vi "RMM_4WIS_RT_DXs_V2_1team.vi"() -> ()   [LabVIEW 2019]
uses:
  <vilib>/Instr/_visa.llb/VISA Set IO Buffer Mask.ctl
  <vilib>/Instr/_visa.llb/VISA Flush IO Buffer Mask.ctl
  <vilib>/Instr/_visa.llb/VISA Configure Serial Port (Instr).vi
  <vilib>/FPGAPlugInAG/myRIO-1900/niLvFpga_Open_myRIO-1900.vi
  <vilib>/rvi/interface/common/dynamic/niFpgaDynamicAddResources.vi
  <vilib>/Utility/error.llb/Error Cluster From Error Code.vi
  <vilib>/rvi/errors/niLvFpgaAdjustHostInterfaceError.vi
  <vilib>/FPGAPlugInAG/Dynamic/niLvFpga_Close_Dynamic.vi
  <vilib>/rvi/interface/nirviOpenFPGA/nirviOpenFPGA.xnode
  FPGA Bitfiles/rmm4wisrobot_FPGATarget_RMM4WISFPGA_VGKxlyhi8sc.lvbitx
  RMM_4WIS_FPGA.vi
  <vilib>/rvi/interface/nirviReadWriteControl/nirviReadWriteControl.xnode
  <vilib>/rvi/interface/nirviCloseFPGA/nirviCloseFPGA.xnode
  <vilib>/rvi/interface/Simulation/niFpgaSimulationCallBeginRW.vi
  NiFpgaLv.dll
panel:
  out "RL_Steer_Feed(deg)":i16
  out "RR_Steer_Feed(deg)":i16
  out "FR_Steer_Feed(deg)":i16
  out "FL_Steer_Feed(deg)":i16
  out "HLV_M/A_Status":u8
  out "K_ZERO_CMD":T1
  out "RIO_Steer_Mode":u8
  out "HLV_NotAlive":bool
  out "HLV_E-Stop":bool
  out "RE_E-Stop":bool
  out "Re_M/A":bool
  out "FR_M1_Curr.MPS":dbl
  out "RL_M2_Curr.MPS":dbl
  out "RR_Steer_Feed":i16
  out "RL_Steer_Feed":i16
  out "FR_Steer_Feed":i16
  out "FL_Steer_Feed":i16
  out "Rear_Data":string
  out "RR_M1_Curr.RPM":i16
  out "RR_M1_Amp":u16
  out "RR_M1_Encoder":i32
  out "RR_M1_Staus":u8
  out "RL_M2_Curr.RPM":i16
  out "RL_M2_Amp":u16
  out "RL_M2_Staus":u8
  out "RL_M2_Encoder":i32
  out "RR_M1_Curr.MPS":dbl
  out "RL_RPM":i16
  out "R_TQ_Off":bool
  out "FL_M1_Curr.MPS":dbl
  out "FR_M2_Encoder":i32
  out "FR_M2_Staus":u8
  out "FR_M2_Amp":u16
  out "FR_M2_Curr.RPM":i16
  out "FL_M1_Staus":u8
  out "FR_RPM":i16
  out "FL_RPM":i16
  out "RR_RPM":i16
  out "FL_M1_Encoder":i32
  out "FL_M1_Amp":u16
  out "FL_M1_Curr.RPM":i16
  out "F_TQ_Off":bool
  out "Front_Data":string
  in  "정지":bool
  # "Front"
  # "Rear"
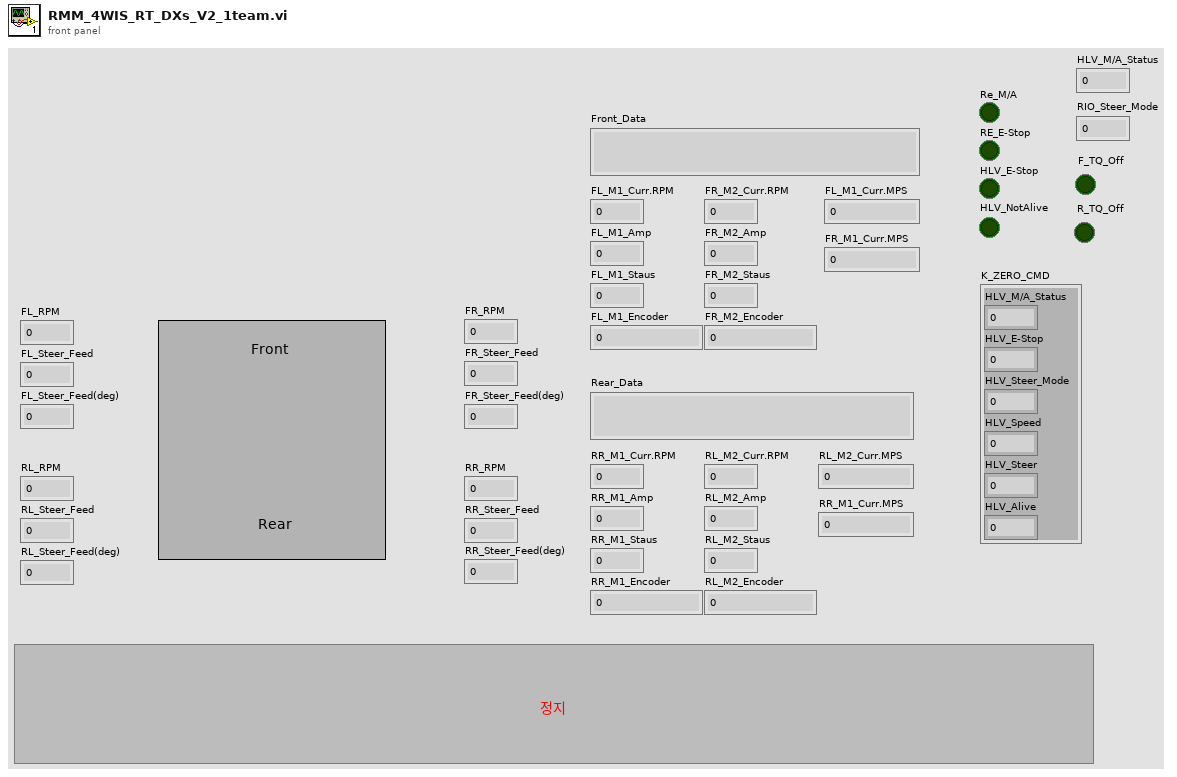
[diagram p1: front panel]
types:
  T1 = cluster{"HLV_M/A_Status":u8, "HLV_E-Stop":u8, "HLV_Steer_Mode":u8, "HLV_Speed":i16, "HLV_Steer":i16, "HLV_Alive":u8}
  T2 = cluster{"RIO_M/A_Status":u8, "RIO_E-Stop":u8, "RIO_Steer_Mode":u8, "RIO_FL_Speed":i16, "RIO_FL_Steer":i16, "RIO_Alive":u8, "RIO_FR_Speed":i16, "RIO_RL_Speed":i16, "RIO_RR_Speed":i16, "RIO_FR_Steer":i16, "RIO_RL_Steer":i16, "RIO_RR_Steer":i16}
  T3 = typedef "VISA Flush IO Buffer Mask.ctl" = u16
  T4 = typedef "VISA Set IO Buffer Mask.ctl" = u16
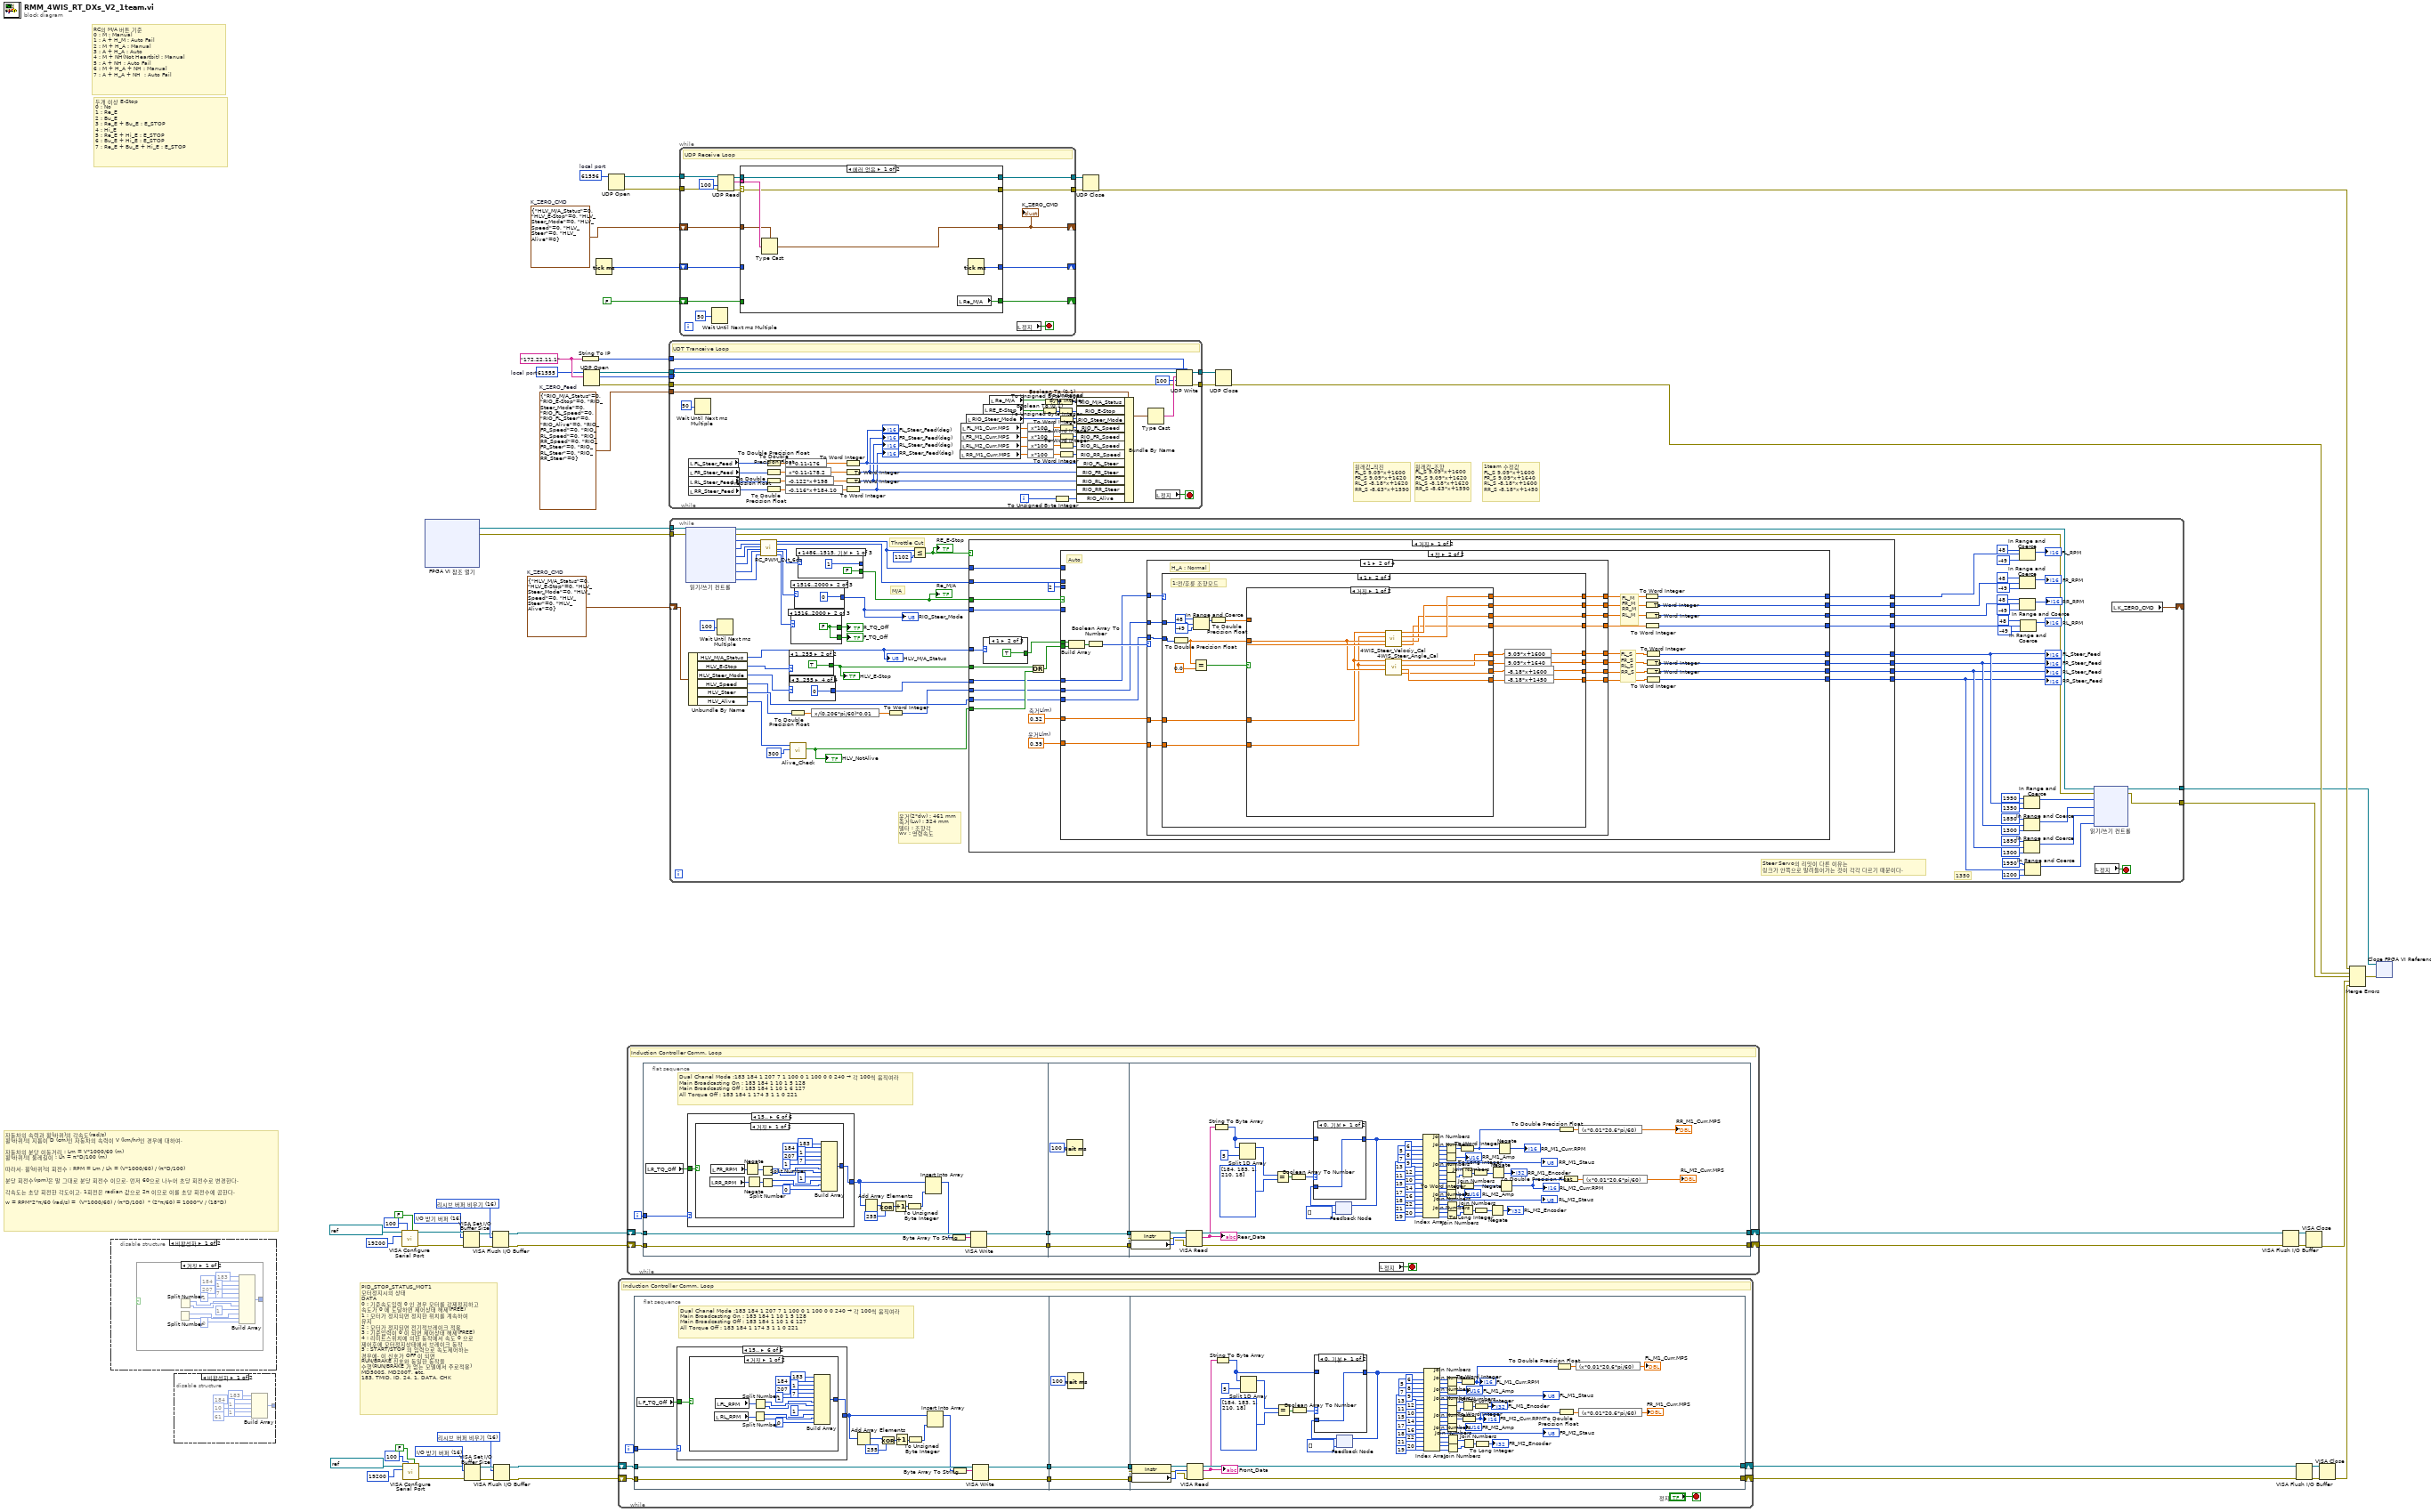
[diagram p0: block diagram]
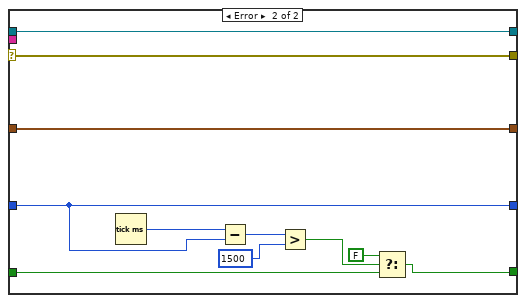
[diagram p2: hidden frame]
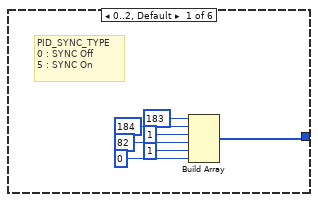
[diagram p3: hidden frame]
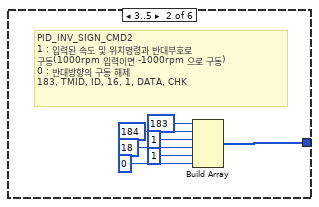
[diagram p4: hidden frame]
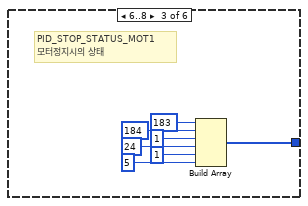
[diagram p5: hidden frame]
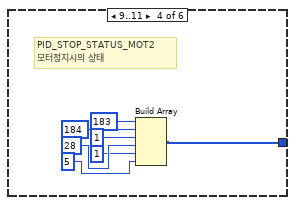
[diagram p6: hidden frame]
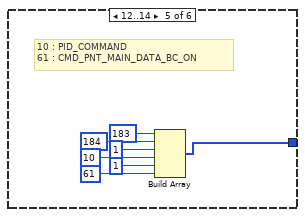
[diagram p7: hidden frame]
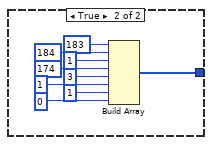
[diagram p8: hidden frame]
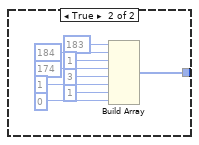
[diagram p11: hidden frame]
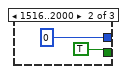
[diagram p13: hidden frame]
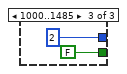
[diagram p14: hidden frame]
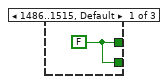
[diagram p15: hidden frame]
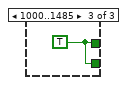
[diagram p16: hidden frame]
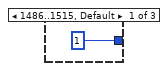
[diagram p17: hidden frame]
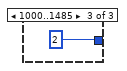
[diagram p18: hidden frame]
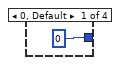
[diagram p19: hidden frame]
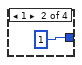
[diagram p20: hidden frame]
diagram:
  w3 = T2 {"RIO_M/A_Status"=0, "RIO_E-Stop"=0, "RIO_Steer_Mode"=0, "RIO_FL_Speed"=0, "RIO_FL_Steer"=0, "RIO_Alive"=0, "RIO_FR_Speed"=0, "RIO_RL_Speed"=0, "RIO_RR_Speed"=0, "RIO_FR_Steer"=0, "RIO_RL_Steer"=0, "RIO_RR_Steer"=0}  # K_ZERO_Feed
  w4 = T1 {"HLV_M/A_Status"=0, "HLV_E-Stop"=0, "HLV_Steer_Mode"=0, "HLV_Speed"=0, "HLV_Steer"=0, "HLV_Alive"=0}  # K_ZERO_CMD
  w12 = u16 61555  # local port
  w13 = "172.22.11.1" ("name")
  w21 = u16 61556  # local port
  w20 = T1 {"HLV_M/A_Status"=0, "HLV_E-Stop"=0, "HLV_Steer_Mode"=0, "HLV_Speed"=0, "HLV_Steer"=0, "HLV_Alive"=0}  # K_ZERO_CMD
  w35 = T3 16 items=["리시브 버퍼 비우기"=16, "전달 버퍼 디바이스에 쓰기"=32, "리시브 버퍼 비우기(I/O 없음)"=64, "전달 버퍼 비우기"=128] ("Mask")
  w34 = T4 16 items=["I/O 받기 버퍼"=16, "I/O 전달 버퍼"=32, "I/O 받기와 전달 버퍼"=48] ("Mask")
  w52 = T3 16 items=["리시브 버퍼 비우기"=16, "전달 버퍼 디바이스에 쓰기"=32, "리시브 버퍼 비우기(I/O 없음)"=64, "전달 버퍼 비우기"=128] ("Mask")
  w53 = T4 16 items=["I/O 받기 버퍼"=16, "I/O 전달 버퍼"=32, "I/O 받기와 전달 버퍼"=48] ("Mask")
  # "원래값_직진\nFL_S 9.09*x+1600\nFR_S 9.09*x+1620\nRL_S -8.18*x+1620\nRR_S -8.63*x+1590"
  # "1team 수정값\nFL_S 9.09*x+1600\nFR_S 9.09*x+1640\nRL_S -8.18*x+1600\nRR_S -8.18*x+1450"
  # "원래값_조향\nFL_S 9.09*x+1600\nFR_S 9.09*x+1620\nRL_S -8.18*x+1620\nRR_S -8.63*x+1590"
  # "PID_STOP_STATUS_MOT1\n모터정지시의 상태\nDATA\n0 : 기준속도입력 0 인 경우 모터를 강제정지하고\n속도가 0 에 도달하면 제어상태 해제(FREE)\n1 : 모터가 정지되면 정지한 위치를 계속하여\n유지\n2 : 모터가 정지되면 전기적브레이크 적용\n3 : 기준입력이 0 이 되면 제어상태 해제(FREE)\n4 : 리미트스위치에 의한 동작에서 속도 0 으로\n제어후에 모터정지상태에서 브레이크 동작\n5 : START/STOP 의 입력으로 속도제어하는\n경우에, 이 신호가 OFF 이 되면\nRUN/BRAKE 신호와 동일한 동작을\n수행(RUN/BRAKE 가 없는 모델에서 주로적용)\nMD500S, MD200T, etc.\n183, TMID, ID, 24, 1, DATA, CHK"
  # "두개 이상 E-Stop\n0 : No\n1 : Re_E\n2 : Bu_E\n3 : Re_E + Bu_E : E_STOP\n4 : Hi_E\n5 : Re_E + Hi_E : E_STOP\n6 : Bu_E + Hi_E : E_STOP\n7 : Re_E + Bu_E + Hi_E : E_STOP"
  # "RC의 M/A 버튼 기준\n0 : M : Manual \n1 : A + H_M : Auto Fail\n2 : M + H_A : Manual\n3 : A + H_A : Auto\n4 : M + NH(Not Heartbit) : Manual\n5 : A + NH : Auto Fail\n6 : M + H_A + NH : Manual\n7 : A + H_A + NH  : Auto Fail"
  # "자동차의 속력과 휠(바퀴)의 각속도(rad/s)\n휠(바퀴)의 지름이 D (cm)인 자동차의 속력이 V (km/hr)인 경우에 대하여,  \n\n자동차의 분당 이동거리 : Lm = V*1000/60 (m)  \n휠(바퀴)의 둘레길이 : Lh = π*D/100 (m)  \n\n따라서, 휠(바퀴)의 회전수 : RPM = Lm / Lh = (V*1000/60) / (π*D/100)  \n\n분당 회전수(rpm)은 말 그대로 분당 회전수 이므로, 먼저 60으로 나누어 초당 회전수로 변경한다.  \n\n각속도는 초당 회전한 각도이고, 1회전은 radian 값으로 2π 이므로 이를 초당 회전수에 곱한다.  \n\nw = RPM*2*π/60 (rad/s) =  (V*1000/60) / (π*D/100)  * (2*π/60) = 1000*V / (18*D)"
  n1 = disable-structure shown="비활성화" {
    frame Disabled {
      n2 = case shown="거짓" {
        selector: _ -> [_ _]
        tunnel: [w64 w73] -> _
        frame False {
          n3 = Split Number() -> (hi(x)=w61:u16, lo(x)=w60:u16)  [unwired: 1 in]
          n4 = Split Number() -> (hi(x)=w63:u16, lo(x)=w62:u16)  [unwired: 1 in]
          n5 = Build Array(u8 183, u8 184, u8 1, u8 207, u8 7, u8 1, w62, w63, u8 1, w60, w61, u8 0) -> (w64:u8[])
        }
        frame True {
          n6 = Build Array(u8 183, u8 184, u8 1, u8 174, u8 3, u8 1, u8 1, u8 0) -> (w73:u8[])
        }
      }
    }
    frame Enabled {
    }
  }
  n7 = disable-structure shown="비활성화" {
    disable-tunnel: [w88 _] -> _
    frame Disabled {
      n8 = Build Array(u8 183, u8 184, u8 1, u8 10, u8 1, u8 61) -> (w88:u8[])
    }
    frame Enabled {
    }
  }
  n9 = call-poly "VISA Configure Serial Port"("VISA resource name"=refnum<visa-resource-name> "ASRL2::INSTR", "timeout (10sec)"=u32 100, "Enable Termination\nChar (T)"=FALSE ("Enable Termination\nChar (T)"), "baud rate (9600)"=u32 19200) -> ("VISA resource name out"=w42:refnum<visa-resource-name>, "error out"=w43:errorcluster)  [unwired: 10 in]
  n10 = call-poly "VISA Configure Serial Port"("VISA resource name"=refnum<visa-resource-name> "ASRL1::INSTR", "timeout (10sec)"=u32 100, "Enable Termination\nChar (T)"=FALSE ("Enable Termination\nChar (T)"), "baud rate (9600)"=u32 19200) -> ("VISA resource name out"=w45:refnum<visa-resource-name>, "error out"=w44:errorcluster)  [unwired: 10 in]
  n11 = xnode "FPGA VI 참조 열기"() -> ("FPGA VI 참조 출력"=w2:refnum<k20>, "에러 출력"=w1:errorcluster)  [unwired: 2 in]
  n12 = VISA Set I/O Buffer Size(VISA resource name=w42, mask (16)=w34, error in (no error)=w43) -> (VISA resource name out=w32:refnum<visa-resource-name>, error out=w33:errorcluster)  [unwired: 1 in]
  n13 = VISA Set I/O Buffer Size(VISA resource name=w45, mask (16)=w53, error in (no error)=w44) -> (VISA resource name out=w55:refnum<visa-resource-name>, error out=w54:errorcluster)  [unwired: 1 in]
  n14 = VISA Flush I/O Buffer(VISA resource name=w32, mask (16)=w35, error in (no error)=w33) -> (VISA resource name out=w36:refnum<visa-resource-name>, error out=w37:errorcluster)
  n15 = VISA Flush I/O Buffer(VISA resource name=w55, mask (16)=w52, error in (no error)=w54) -> (VISA resource name out=w51:refnum<visa-resource-name>, error out=w50:errorcluster)
  n16 = String To IP(1:w13) -> (0:w14:u32)
  n17 = UDP Open(10:w13, 11:w12) -> (port=w15:refnum<k16>, 0:w16:errorcluster, 2:w17:u16)  [unwired: 3 in]
  n18 = Tick Count (ms)() -> (millisecond timer value=w24:u32)
  n19 = UDP Open(11:w21) -> (port=w22:refnum<k16>, 0:w23:errorcluster)  [unwired: 4 in, 1 out]
  n20 = while {
    shift-right: [w91] -> w49
    shift-left: w51 -> [w97]
    shift-right: [w90] -> w48
    shift-left: w50 -> [w96]
    i -> [w89]
    stop <- "정지" stop-if-true
    # "Induction Controller Comm. Loop"
    n21 = flat-sequence {
      tunnel: [w110] -> w94
      tunnel: [w109] -> w92
      tunnel: w97 -> [w112]
      tunnel: w96 -> [w111]
      tunnel: w89 -> [w107]
      tunnel: [w176] -> w95
      tunnel: w94 -> [w176]
      tunnel: [w175] -> w93
      tunnel: w92 -> [w175]
      tunnel: w95 -> [w245]
      tunnel: w93 -> [w244]
      tunnel: [w247] -> w91
      tunnel: [w246] -> w90
      frame #0 {
        # "Dual Chanel Mode :183 184 1 207 7 1 100 0 1 100 0 0 240 → 각 100씩 움직여라\nMain Broadcasting On : 183 184 1 10 1 5 128\nMain Broadcasting Off : 183 184 1 10 1 6 127\nAll Torque Off : 183 184 1 174 3 1 1 0 221"
        n22 = local read "F_TQ_Off"() -> (w99:bool)
        n23 = case shown="15.." w107 {
          tunnel: [w113 w120 w127 w134 w141 w149] -> w100
          tunnel: w99 -> [_ _ _ _ _ w148]
          frame 0..2, Default {
            # "PID_SYNC_TYPE\n0 : SYNC Off\n5 : SYNC On"
            n24 = Build Array(u8 183, u8 184, u8 1, u8 82, u8 1, u8 0) -> (w113:u8[])
          }
          frame 3..5 {
            # "PID_INV_SIGN_CMD2\n1 : 모터 2 에 관한 명령으로 입력된 속도 및\n위치명령과 반대부호로 구동\n(1000rpm 입력이면 -1000rpm 으로 구동)\n0 : 반대방향의 구동 해제"
            n25 = Build Array(u8 183, u8 184, u8 1, u8 18, u8 1, u8 0) -> (w120:u8[])
          }
          frame 6..8 {
            # "PID_STOP_STATUS_MOT1\n모터정지시의 상태"
            n26 = Build Array(u8 183, u8 184, u8 1, u8 24, u8 1, u8 5) -> (w127:u8[])
          }
          frame 9..11 {
            # "PID_STOP_STATUS_MOT2\n모터정지시의 상태"
            n27 = Build Array(u8 183, u8 184, u8 1, u8 28, u8 1, u8 5) -> (w134:u8[])
          }
          frame 12..14 {
            # "10 : PID_COMMAND\n61 : CMD_PNT_MAIN_DATA_BC_ON"
            n28 = Build Array(u8 183, u8 184, u8 1, u8 10, u8 1, u8 61) -> (w141:u8[])
          }
          frame 15.. {
            n29 = case shown="거짓" w148 {
              tunnel: [w156 w165] -> w149
              frame False {
                n30 = local read "RL_RPM"() -> (w150:i16)
                n31 = local read "FL_RPM"() -> (w151:i16)
                n32 = Split Number(x=w150) -> (hi(x)=w153:u8, lo(x)=w152:u8)
                n33 = Split Number(x=w151) -> (hi(x)=w155:u8, lo(x)=w154:u8)
                n34 = Build Array(u8 183, u8 184, u8 1, u8 207, u8 7, u8 1, w154, w155, u8 1, w152, w153, u8 0) -> (w156:u8[])
              }
              frame True {
                n35 = Build Array(u8 183, u8 184, u8 1, u8 174, u8 3, u8 1, u8 1, u8 0) -> (w165:u8[])
              }
            }
          }
        }
        n36 = Add Array Elements(numeric array=w100) -> (sum=w104:u8)
        n37 = Exclusive Or(1:u8 255 ("y"), 2:w104) -> (0:w105:u8)
        n38 = Increment(x=w105) -> (x+1=w106:u8)
        n39 = To Unsigned Byte Integer(number=w106) -> (unsigned 8bit integer=w102:u8)
        n40 = Insert Into Array(array=w100, new element=w102) -> (w101:u8[])  [unwired: 1 in]
        n41 = Byte Array To String(unsigned byte array=w101) -> (string=w108:string)
        n42 = VISA Write(VISA resource name=w112, write buffer=w108, error in (no error)=w111) -> (VISA resource name out=w110:refnum<visa-resource-name>, error out=w109:errorcluster)  [unwired: 1 out]
      }
      frame #1 {
        n43 = Wait (ms)(milliseconds to wait=u32 100 ("대기 시간 (ms)")) -> ()  [unwired: 1 out]
      }
      frame #2 {
        n44 = property class="Instr"(reference=w245, error in=w244) -> (reference out=w243:refnum<visa-resource-name>, error out=w241:errorcluster, "Serial Settings:Number of Bytes at Serial Port"=w242:u32)
        n45 = VISA Read(VISA resource name=w243, byte count=w242, error in (no error)=w241) -> (VISA resource name out=w247:refnum<visa-resource-name>, read buffer=w240:string, error out=w246:errorcluster)  [unwired: 1 out]
        "Front_Data" <- w240
        n46 = String To Byte Array(string=w240) -> (unsigned byte array=w239:u8[])
        n47 = Split 1D Array(array=w239, index=5) -> (first subarray=w235:u8[])  [unwired: 1 out]
        n48 = Equal?(x=w235, y=u8[] [184, 183, 1, 210, 18]) -> (x = y?=w237:bool[])
        n49 = Boolean Array To Number(Boolean array=w237) -> (number=w236:u32)
        n50 = feedback #1(u8[] [] ("unsigned byte array")) -> (w183:u8[])
        n51 = case shown="0, 기본" w236 {
          tunnel: w239 -> [_ w249]
          tunnel: [w248 w249] -> w184
          tunnel: w183 -> [w248 _]
          frame 0, Default {
          }
          frame 31 {
          }
        }
        n52 = feedback-in #1(w184) -> ()
        n53 = Index Array(array=w184, index #1=6, index #2=5, index #3=8, index #4=7, index #5=9, index #6=13, index #7=12, index #8=11, index #9=10, index #10=15, index #11=14, index #12=17, index #13=16, index #14=18, index #15=22, index #16=21, index #17=20, index #18=19) -> (element #1=w232:u8, element #2=w231:u8, element #3=w229:u8, element #4=w227:u8, element #5=→"FL_M1_Staus":u8, element #6=w226:u8, element #7=w225:u8, element #8=w224:u8, element #9=w223:u8, element #10=w217:u8, element #11=w216:u8, element #12=w214:u8, element #13=w213:u8, element #14=→"FR_M2_Staus":u8, element #15=w207:u8, element #16=w206:u8, element #17=w205:u8, element #18=w204:u8)
        n54 = Join Numbers(hi=w232, lo=w231) -> ((hi.lo)=w230:u16)
        n55 = Join Numbers(hi=w229, lo=w227) -> ((hi.lo)=→"FL_M1_Amp":u16)
        n56 = Join Numbers(hi=w226, lo=w225) -> ((hi.lo)=w219:u16)
        n57 = Join Numbers(hi=w224, lo=w223) -> ((hi.lo)=w218:u16)
        n58 = Join Numbers(hi=w217, lo=w216) -> ((hi.lo)=w215:u16)
        n59 = Join Numbers(hi=w214, lo=w213) -> ((hi.lo)=→"FR_M2_Amp":u16)
        n60 = Join Numbers(hi=w207, lo=w206) -> ((hi.lo)=w210:u16)
        n61 = Join Numbers(hi=w205, lo=w204) -> ((hi.lo)=w203:u16)
        n62 = To Word Integer(number=w230) -> (16bit integer=w182:i16)
        "FL_M1_Curr.RPM" <- w182
        n63 = Join Numbers(hi=w219, lo=w218) -> ((hi.lo)=w222:u32)
        n64 = To Word Integer(number=w215) -> (16bit integer=w177:i16)
        "FR_M2_Curr.RPM" <- w177
        n65 = Join Numbers(hi=w210, lo=w203) -> ((hi.lo)=w208:u32)
        n66 = To Long Integer(number=w222) -> (32bit integer=→"FL_M1_Encoder":i32)
        n67 = To Long Integer(number=w208) -> (32bit integer=→"FR_M2_Encoder":i32)
        n68 = To Double Precision Float(number=w182) -> (double precision float=w180:dbl)
        n69 = To Double Precision Float(number=w177) -> (double precision float=w179:dbl)
        n70 = expression code="(x*0.01*20.6*pi/60)"(w180) -> (→"FL_M1_Curr.MPS":dbl)
        n71 = expression code="(x*0.01*20.6*pi/60)"(w179) -> (→"FR_M1_Curr.MPS":dbl)
      }
    }
  }
  n72 = while {
    shift-right: [w253] -> w38
    shift-left: w36 -> [w259]
    shift-right: [w252] -> w39
    shift-left: w37 -> [w258]
    i -> [w251]
    stop <- w250 stop-if-true
    # "Induction Controller Comm. Loop"
    n73 = flat-sequence {
      tunnel: [w271] -> w256
      tunnel: [w270] -> w254
      tunnel: w259 -> [w273]
      tunnel: w258 -> [w272]
      tunnel: w251 -> [w268]
      tunnel: [w339] -> w257
      tunnel: w256 -> [w339]
      tunnel: [w338] -> w255
      tunnel: w254 -> [w338]
      tunnel: w257 -> [w412]
      tunnel: w255 -> [w411]
      tunnel: [w414] -> w253
      tunnel: [w413] -> w252
      frame #0 {
        # "Dual Chanel Mode :183 184 1 207 7 1 100 0 1 100 0 0 240 → 각 100씩 움직여라\nMain Broadcasting On : 183 184 1 10 1 5 128\nMain Broadcasting Off : 183 184 1 10 1 6 127\nAll Torque Off : 183 184 1 174 3 1 1 0 221"
        n74 = local read "R_TQ_Off"() -> (w260:bool)
        n75 = case shown="15.." w268 {
          tunnel: [w274 w281 w288 w295 w302 w310] -> w261
          tunnel: w260 -> [_ _ _ _ _ w309]
          frame 0..2, Default {
            # "PID_SYNC_TYPE\n0 : SYNC Off\n5 : SYNC On"
            n76 = Build Array(u8 183, u8 184, u8 1, u8 82, u8 1, u8 0) -> (w274:u8[])
          }
          frame 3..5 {
            # "PID_INV_SIGN_CMD2\n1 : 입력된 속도 및 위치명령과 반대부호로\n구동(1000rpm 입력이면 -1000rpm 으로 구동)\n0 : 반대방향의 구동 해제\n183, TMID, ID, 16, 1, DATA, CHK"
            n77 = Build Array(u8 183, u8 184, u8 1, u8 18, u8 1, u8 0) -> (w281:u8[])
          }
          frame 6..8 {
            # "PID_STOP_STATUS_MOT1\n모터정지시의 상태"
            n78 = Build Array(u8 183, u8 184, u8 1, u8 24, u8 1, u8 5) -> (w288:u8[])
          }
          frame 9..11 {
            # "PID_STOP_STATUS_MOT2\n모터정지시의 상태"
            n79 = Build Array(u8 183, u8 184, u8 1, u8 28, u8 1, u8 5) -> (w295:u8[])
          }
          frame 12..14 {
            # "10 : PID_COMMAND\n61 : CMD_PNT_MAIN_DATA_BC_ON"
            n80 = Build Array(u8 183, u8 184, u8 1, u8 10, u8 1, u8 61) -> (w302:u8[])
          }
          frame 15.. {
            n81 = case shown="거짓" w309 {
              tunnel: [w319 w328] -> w310
              frame False {
                n82 = local read "RR_RPM"() -> (w314:i16)
                n83 = local read "FR_RPM"() -> (w313:i16)
                n84 = Negate(x=w313) -> (-x=w312:i16)
                n85 = Negate(x=w314) -> (-x=w311:i16)
                n86 = Split Number(x=w311) -> (hi(x)=w316:u8, lo(x)=w315:u8)
                n87 = Split Number(x=w312) -> (hi(x)=w318:u8, lo(x)=w317:u8)
                n88 = Build Array(u8 183, u8 184, u8 1, u8 207, u8 7, u8 1, w317, w318, u8 1, w315, w316, u8 0) -> (w319:u8[])
              }
              frame True {
                n89 = Build Array(u8 183, u8 184, u8 1, u8 174, u8 3, u8 1, u8 1, u8 0) -> (w328:u8[])
              }
            }
          }
        }
        n90 = Add Array Elements(numeric array=w261) -> (sum=w265:u8)
        n91 = Exclusive Or(1:u8 255 ("y"), 2:w265) -> (0:w266:u8)
        n92 = Increment(x=w266) -> (x+1=w267:u8)
        n93 = To Unsigned Byte Integer(number=w267) -> (unsigned 8bit integer=w263:u8)
        n94 = Insert Into Array(array=w261, new element=w263) -> (w262:u8[])  [unwired: 1 in]
        n95 = Byte Array To String(unsigned byte array=w262) -> (string=w269:string)
        n96 = VISA Write(VISA resource name=w273, write buffer=w269, error in (no error)=w272) -> (VISA resource name out=w271:refnum<visa-resource-name>, error out=w270:errorcluster)  [unwired: 1 out]
      }
      frame #1 {
        n97 = Wait (ms)(milliseconds to wait=u32 100 ("대기 시간 (ms)")) -> ()  [unwired: 1 out]
      }
      frame #2 {
        n98 = property class="Instr"(reference=w412, error in=w411) -> (reference out=w410:refnum<visa-resource-name>, error out=w408:errorcluster, "Serial Settings:Number of Bytes at Serial Port"=w409:u32)
        n99 = VISA Read(VISA resource name=w410, byte count=w409, error in (no error)=w408) -> (VISA resource name out=w414:refnum<visa-resource-name>, read buffer=w407:string, error out=w413:errorcluster)  [unwired: 1 out]
        "Rear_Data" <- w407
        n100 = String To Byte Array(string=w407) -> (unsigned byte array=w406:u8[])
        n101 = Split 1D Array(array=w406, index=5) -> (first subarray=w402:u8[])  [unwired: 1 out]
        n102 = Equal?(x=w402, y=u8[] [184, 183, 1, 210, 18]) -> (x = y?=w404:bool[])
        n103 = Boolean Array To Number(Boolean array=w404) -> (number=w403:u32)
        n104 = feedback #2(u8[] [] ("unsigned byte array")) -> (w352:u8[])
        n105 = case shown="0, 기본" w403 {
          tunnel: w406 -> [_ w416]
          tunnel: [w415 w416] -> w353
          tunnel: w352 -> [w415 _]
          frame 0, Default {
          }
          frame 31 {
          }
        }
        n106 = feedback-in #2(w353) -> ()
        n107 = Index Array(array=w353, index #1=6, index #2=5, index #3=8, index #4=7, index #5=9, index #6=13, index #7=12, index #8=11, index #9=10, index #10=15, index #11=14, index #12=17, index #13=16, index #14=18, index #15=22, index #16=21, index #17=20, index #18=19) -> (element #1=w399:u8, element #2=w398:u8, element #3=w396:u8, element #4=w394:u8, element #5=→"RR_M1_Staus":u8, element #6=w393:u8, element #7=w392:u8, element #8=w391:u8, element #9=w390:u8, element #10=w385:u8, element #11=w384:u8, element #12=w382:u8, element #13=w381:u8, element #14=→"RL_M2_Staus":u8, element #15=w376:u8, element #16=w375:u8, element #17=w374:u8, element #18=w373:u8)
        n108 = Join Numbers(hi=w399, lo=w398) -> ((hi.lo)=w397:u16)
        n109 = Join Numbers(hi=w396, lo=w394) -> ((hi.lo)=→"RR_M1_Amp":u16)
        n110 = Join Numbers(hi=w393, lo=w392) -> ((hi.lo)=w387:u16)
        n111 = Join Numbers(hi=w391, lo=w390) -> ((hi.lo)=w386:u16)
        n112 = Join Numbers(hi=w385, lo=w384) -> ((hi.lo)=w383:u16)
        n113 = Join Numbers(hi=w382, lo=w381) -> ((hi.lo)=→"RL_M2_Amp":u16)
        n114 = Join Numbers(hi=w376, lo=w375) -> ((hi.lo)=w378:u16)
        n115 = Join Numbers(hi=w374, lo=w373) -> ((hi.lo)=w372:u16)
        n116 = To Word Integer(number=w397) -> (16bit integer=w346:i16)
        n117 = Join Numbers(hi=w387, lo=w386) -> ((hi.lo)=w389:u32)
        n118 = To Word Integer(number=w383) -> (16bit integer=w347:i16)
        n119 = Join Numbers(hi=w378, lo=w372) -> ((hi.lo)=w377:u32)
        n120 = To Long Integer(number=w389) -> (32bit integer=w350:i32)
        n121 = To Long Integer(number=w377) -> (32bit integer=w349:i32)
        n122 = Negate(x=w349) -> (-x=→"RL_M2_Encoder":i32)
        n123 = Negate(x=w350) -> (-x=→"RR_M1_Encoder":i32)
        n124 = Negate(x=w346) -> (-x=→"RR_M1_Curr.RPM":i16)
        n125 = Negate(x=w347) -> (-x=w341:i16)
        "RL_M2_Curr.RPM" <- w341
        n126 = To Double Precision Float(number=w346) -> (double precision float=w351:dbl)
        n127 = To Double Precision Float(number=w341) -> (double precision float=w348:dbl)
        n128 = expression code="(x*0.01*20.6*pi/60)"(w351) -> (→"RR_M1_Curr.MPS":dbl)
        n129 = expression code="(x*0.01*20.6*pi/60)"(w348) -> (→"RL_M2_Curr.MPS":dbl)
      }
    }
    n130 = local read "정지"() -> (w250:bool)
  }
  n131 = while {
    tunnel: w3 -> [w455]
    tunnel: w14 -> [w463]
    tunnel: w15 -> [w465]
    tunnel: w16 -> [w448]
    tunnel: w17 -> [w464]
    tunnel: [w451] -> w18
    tunnel: [w450] -> w19
    i -> [w454]
    stop <- w449 stop-if-true
    # "UDT Tranceive Loop"
    n132 = local read "FL_Steer_Feed"() -> (w431:i16)
    n133 = local read "FR_Steer_Feed"() -> (w426:i16)
    n134 = local read "RL_Steer_Feed"() -> (w423:i16)
    n135 = local read "RR_Steer_Feed"() -> (w422:i16)
    n136 = Wait Until Next ms Multiple(millisecond multiple=u32 50) -> ()  [unwired: 1 out]
    n137 = To Double Precision Float(number=w431) -> (double precision float=w432:dbl)
    n138 = To Double Precision Float(number=w426) -> (double precision float=w427:dbl)
    n139 = To Double Precision Float(number=w423) -> (double precision float=w421:dbl)
    n140 = To Double Precision Float(number=w422) -> (double precision float=w425:dbl)
    n141 = expression code="x*0.11-176"(w432) -> (w430:dbl)
    n142 = expression code="x*0.11-178.2"(w427) -> (w428:dbl)
    n143 = expression code="-0.122*x+198"(w421) -> (w420:dbl)
    n144 = expression code="-0.116*x+184.10"(w425) -> (w424:dbl)
    n145 = To Word Integer(number=w430) -> (16bit integer=w429:i16)
    "FL_Steer_Feed(deg)" <- w429
    n146 = To Word Integer(number=w428) -> (16bit integer=w419:i16)
    "FR_Steer_Feed(deg)" <- w419
    n147 = To Word Integer(number=w420) -> (16bit integer=w418:i16)
    "RL_Steer_Feed(deg)" <- w418
    n148 = To Word Integer(number=w424) -> (16bit integer=w417:i16)
    "RR_Steer_Feed(deg)" <- w417
    n149 = local read "RR_M1_Curr.MPS"() -> (w433:dbl)
    n150 = local read "FR_M1_Curr.MPS"() -> (w435:dbl)
    n151 = local read "RL_M2_Curr.MPS"() -> (w434:dbl)
    n152 = local read "FL_M1_Curr.MPS"() -> (w442:dbl)
    n153 = local read "RIO_Steer_Mode"() -> (w444:u8)
    n154 = local read "RE_E-Stop"() -> (w462:bool)
    n155 = local read "Re_M/A"() -> (w445:bool)
    n156 = expression code="x*100"(w442) -> (w446:dbl)
    n157 = expression code="x*100"(w435) -> (w441:dbl)
    n158 = expression code="x*100"(w434) -> (w436:dbl)
    n159 = expression code="x*100"(w433) -> (w437:dbl)
    n160 = Boolean To (0,1)(Boolean=w462) -> (0, 1=w458:i16)
    n161 = Boolean To (0,1)(Boolean=w445) -> (0, 1=w457:i16)
    n162 = To Unsigned Byte Integer(number=w454) -> (unsigned 8bit integer=w443:u8)
    n163 = To Unsigned Byte Integer(number=w457) -> (unsigned 8bit integer=w456:u8)
    n164 = To Unsigned Byte Integer(number=w458) -> (unsigned 8bit integer=w459:u8)
    n165 = To Unsigned Byte Integer(number=w444) -> (unsigned 8bit integer=w460:u8)
    n166 = To Word Integer(number=w446) -> (16bit integer=w461:i16)
    n167 = To Word Integer(number=w441) -> (16bit integer=w438:i16)
    n168 = To Word Integer(number=w436) -> (16bit integer=w439:i16)
    n169 = To Word Integer(number=w437) -> (16bit integer=w440:i16)
    n170 = Bundle By Name(cluster=w455, "RIO_M/A_Status"=w456, "RIO_E-Stop"=w459, "RIO_Steer_Mode"=w460, "RIO_FL_Speed"=w461, "RIO_FR_Speed"=w438, "RIO_RL_Speed"=w439, "RIO_RR_Speed"=w440, "RIO_FL_Steer"=w429, "RIO_FR_Steer"=w419, "RIO_RL_Steer"=w418, "RIO_RR_Steer"=w417, "RIO_Alive"=w443) -> (w453:T2)
    n171 = Type Cast(x=w453) -> (*(type *) &x=w452:string)  [unwired: 1 in]
    n172 = local read "정지"() -> (w449:bool)
    n173 = UDP Write(address=w463, port or service name=w464, connection ID=w465, data in=w452, 8:w448, 9:100 ("timeout ms (25000)")) -> (error out=w450:errorcluster, 3:w451:refnum<k16>)
  }
  n174 = while {
    tunnel: w2 -> [w535]
    tunnel: w1 -> [w534]
    tunnel: [w538] -> w6
    tunnel: [w537] -> w7
    shift-right: [w499] -> _
    shift-left: w4 -> [w509]
    stop <- w536 stop-if-true
    # "1350"
    # "윤거(2*dw) : 461 mm\n축거(Lw) : 324 mm\n델타 : 조향각\nwv : 명령속도"
    # "M/A"
    # "Throttle Cut"
    # "Steer Servo의 리밋이 다른 이유는\n링크가 안쪽으로 말려들어가는 것이 각각 다르기 때문이다."
    n175 = xnode "읽기/쓰기 컨트롤"("FPGA VI 참조 입력"=w535, "에러 입력"=w534) -> ("FPGA VI 참조 출력"=w533:refnum<k20>, "에러 출력"=w532:errorcluster, "RC_Port0(Tick)"=w531:u32, "RC_Port1(Tick)"=w530:u32, "RC_Port2(Tick)"=w529:u32, "RC_Port3(Tick)"=w528:u32, "RC_Port4(Tick)"=w527:u32, "RC_Port5(Tick)"=w526:u32)
    n176 = Unbundle By Name(w509) -> ("HLV_M/A_Status"=w477:u8, "HLV_E-Stop"=w508:u8, "HLV_Steer_Mode"=w503:u8, "HLV_Speed"=w485:i16, "HLV_Steer"=w506:i16, "HLV_Alive"=w504:u8)
    "HLV_M/A_Status" <- w477
    n177 = Wait Until Next ms Multiple(millisecond multiple=u32 100) -> ()  [unwired: 1 out]
    n178 = call "RC_PWM_Cvt_6ch.vi"("RC_Port0_In"=w531, "RC_Port1_In"=w530, "RC_Port2_In"=w529, "RC_Port3_In"=w528, "RC_Port4_In"=w527, "RC_Port5_In"=w526) -> ("Throttle"=w501:u16, "Aileron"=w512:u16, "S/W B"=w476:u16, "S/W C"=w481:u16, "S/W D"=w480:u16)  [unwired: 8 in, 1 out]
    n179 = case shown="1..255" w508 {
      tunnel: [FALSE TRUE] -> w507
      frame 0, Default {
      }
      frame 1..255 {
      }
    }
    "HLV_E-Stop" <- w507
    n180 = case shown="3..255" w503 {
      tunnel: [u8 0 u8 1 u8 2 u8 0] -> w502
      frame 0, Default {
      }
      frame 1 {
      }
      frame 2 {
      }
      frame 3..255 {
      }
    }
    n181 = To Double Precision Float(number=w485) -> (double precision float=w484:dbl)
    n182 = call "Alive_Check.vi"("Timeout_msec"=u32 300, "Alv_cnt"=w504) -> ("Timeout"=w500:bool)  [unwired: 8 in, 1 out]
    "HLV_NotAlive" <- w500
    n183 = case shown="1516..2000" w480 {
      tunnel: [w545 w546 w547] -> w479
      tunnel: [w545 w546 w547] -> w478
      frame 1486..1515, Default {
        w545 = FALSE
      }
      frame 1516..2000 {
        w546 = FALSE
      }
      frame 1000..1485 {
        w547 = TRUE
      }
    }
    "R_TQ_Off" <- w479
    "F_TQ_Off" <- w478
    n184 = case shown="1516..2000" w481 {
      tunnel: [u8 1 u8 0 u8 2] -> w486
      frame 1486..1515, Default {
      }
      frame 1516..2000 {
      }
      frame 1000..1485 {
      }
    }
    "RIO_Steer_Mode" <- w486
    n185 = case shown="1486..1515, 기본" w476 {
      tunnel: [u8 1 u8 0 u8 2] -> _
      tunnel: [FALSE TRUE FALSE] -> w467
      frame 1486..1515, Default {
      }
      frame 1516..2000 {
      }
      frame 1000..1485 {
      }
    }
    "Re_M/A" <- w467
    n186 = expression code="x/(0.206*pi/60)*0.01"(w484) -> (w483:dbl)
    n187 = To Word Integer(number=w483) -> (16bit integer=w482:i16)
    n188 = Less Or Equal?(x=w501, y=u16 1102) -> (x <= y?=w510:bool)
    "RE_E-Stop" <- w510
    n189 = case shown="거짓" w510 {
      tunnel: w512 -> [w576 _]
      tunnel: w467 -> [w578 _]
      tunnel: w477 -> [w579 _]
      tunnel: w507 -> [w573 _]
      tunnel: w482 -> [w570 _]
      tunnel: w506 -> [w569 _]
      tunnel: w502 -> [w560 _]
      tunnel: w501 -> [w577 _]
      tunnel: w500 -> [w574 _]
      tunnel: [w571 w856] -> w471
      tunnel: w486 -> [w568 _]
      tunnel: [w567 w855] -> w475
      tunnel: [w566 w854] -> w474
      tunnel: [w565 w853] -> w473
      tunnel: [w564 w852] -> w472
      tunnel: [w563 w856] -> w470
      tunnel: [w562 w856] -> w469
      tunnel: [w561 w856] -> w468
      frame False {
        w559 = 0.39  # 윤거L(m)
        w558 = 0.32  # 축거L(m)
        n190 = case shown="1" w579 {
          tunnel: [FALSE TRUE FALSE] -> w575
          frame 0, Default {
          }
          frame 1 {
          }
          frame 2..255 {
          }
        }
        n191 = Or(x=w573, y=w574) -> (x .or. y?=w572:bool)
        n192 = case shown="참" w578 {
          tunnel: w577 -> [w582 _]
          tunnel: w576 -> [w601 _]
          tunnel: w575 -> [_ w731]
          tunnel: w572 -> [_ w730]
          tunnel: [w603 w720] -> w571
          tunnel: w570 -> [_ w727]
          tunnel: w569 -> [_ w726]
          tunnel: w568 -> [w602 _]
          tunnel: [w587 w725] -> w567
          tunnel: [w586 w724] -> w566
          tunnel: [w585 w723] -> w565
          tunnel: [w584 w722] -> w564
          tunnel: [w594 w719] -> w563
          tunnel: [w593 w718] -> w562
          tunnel: [w592 w717] -> w561
          tunnel: w560 -> [_ w721]
          tunnel: u16 2 -> [w583 _]
          tunnel: w559 -> [w580 w708]
          tunnel: w558 -> [w581 w707]
          frame False {
            # "조향 서보모터 : -18~18 deg \n(-는 좌회전) 1900 ~ 1100"
            # "Manual"
            n193 = case shown="2" w583 {
              tunnel: w582 -> [w604 w614 w623]
              tunnel: [w605 w613 w622] -> w598
              frame 0, Default {
                n194 = case shown="1470..1540, 기본" w604 {
                  selector: w604 -> [w608 _ w611]
                  tunnel: [w606 0.0 w610] -> w605
                  frame 1000..1469 {
                    # "모터 RPM 제어 : -10 ~ 0\n1100 ~ 1492"
                    n195 = To Double Precision Float(number=w608) -> (double precision float=w607:dbl)
                    n196 = expression code="0.02551*x-38.06122"(w607) -> (w606:dbl)
                  }
                  frame 1470..1540, Default {
                  }
                  frame 1541..2000 {
                    # "Speed"
                    # "모터 RPM 제어 : 0~10\n1492 ~ 1900"
                    n197 = To Double Precision Float(number=w611) -> (double precision float=w612:dbl)
                    n198 = expression code="0.02451*x-36.5686"(w612) -> (w610:dbl)
                  }
                }
              }
              frame 1 {
                n199 = case shown="1531..2000" w614 {
                  selector: w614 -> [w617 _ w620]
                  tunnel: [w615 0.0 w619] -> w613
                  frame 1000..1469 {
                    # "모터 RPM 제어 : -20 ~ 0\n1100 ~ 1492"
                    n200 = To Double Precision Float(number=w617) -> (double precision float=w616:dbl)
                    n201 = expression code="0.05102*x-76.1224"(w616) -> (w615:dbl)
                  }
                  frame 1470..1530, Default {
                  }
                  frame 1531..2000 {
                    # "Speed"
                    # "모터 RPM 제어 : 0~20\n1492 ~ 1900"
                    n202 = To Double Precision Float(number=w620) -> (double precision float=w621:dbl)
                    n203 = expression code="0.04901*x-73.1372"(w621) -> (w619:dbl)
                  }
                }
              }
              frame 2 {
                n204 = case shown="1541..2000" w623 {
                  selector: w623 -> [w626 _ w629]
                  tunnel: [w624 0.0 w628] -> w622
                  frame 1000..1469 {
                    # "모터 RPM 제어 : -30 ~ 0\n1100 ~ 1492"
                    n205 = To Double Precision Float(number=w626) -> (double precision float=w625:dbl)
                    n206 = expression code="0.07653*x-114.1837"(w625) -> (w624:dbl)
                  }
                  frame 1470..1540, Default {
                  }
                  frame 1541..2000 {
                    # "Speed"
                    # "모터 RPM 제어 : 0~30\n1492 ~ 1900"
                    n207 = To Double Precision Float(number=w629) -> (double precision float=w630:dbl)
                    n208 = expression code="0.0736*x-109.706"(w630) -> (w628:dbl)
                  }
                }
              }
            }
            n209 = case shown="1516..2000" w601 {
              selector: w601 -> [w633 _ w635]
              tunnel: [w631 0.0 w636] -> w600
              frame 1000..1485 {
                # "우회전"
                n210 = To Double Precision Float(number=w633) -> (double precision float=w632:dbl)
                n211 = expression code="-0.045*x+67.5"(w632) -> (w631:dbl)
              }
              frame 1486..1515, Default {
                (unwired) 1
                # "중립"
              }
              frame 1516..2000 {
                (unwired) 2
                # "좌회전"
                n212 = To Double Precision Float(number=w635) -> (double precision float=w637:dbl)
                n213 = expression code="-0.045*x+67.5"(w637) -> (w636:dbl)
              }
            }
            n214 = case shown="2" w602 {
              tunnel: w600 -> [w640 w671 _]
              tunnel: [w654 w685 1940.0] -> w591
              tunnel: [w653 w684 1300.0] -> w590
              tunnel: [w652 w683 1300.0] -> w589
              tunnel: [w651 w682 1950.0] -> w588
              tunnel: [w648 w680 w701] -> w599
              tunnel: w598 -> [w649 w681 w701]
              tunnel: [w647 w679 w702] -> w597
              tunnel: [w646 w678 w700] -> w596
              tunnel: [w645 w677 w701] -> w595
              tunnel: w581 -> [w639 w670 _]
              tunnel: w580 -> [w638 w669 _]
              frame 0, Default {
                # "FL_M\nFR_M\nRR_M\nRL_M"
                # "FL_S\nFR_S\nRL_S\nRR_S"
                # "Deg"
                # "-22~22deg 기준 \n각 서보 출력값의 직선방정식"
                # "전륜 제어"
                n215 = Equal To 0?(x=w640) -> (x = 0?=w650:bool)
                n216 = case shown="거짓" w650 {
                  tunnel: w640 -> [w663 _]
                  tunnel: [w662 w668] -> w647
                  tunnel: [w661 w668] -> w648
                  tunnel: [w660 w668] -> w646
                  tunnel: [w659 w668] -> w645
                  tunnel: [w657 w667] -> w644
                  tunnel: [w658 w667] -> w643
                  tunnel: [w655 w667] -> w642
                  tunnel: [w656 w667] -> w641
                  tunnel: w649 -> [w664 w668]
                  tunnel: w639 -> [w666 _]
                  tunnel: w638 -> [w665 _]
                  frame False {
                    n217 = call "Ackermann_Steer_Angle_Cal.vi"("축거L(m)"=w666, "윤거W(m)"=w665, "조향각(deg)"=w663) -> ("FR_조향각(deg)"=w658:dbl, "FL_조향각(deg)"=w657:dbl, "RR_조향각(deg)"=w656:dbl, "RL_조향각(deg)"=w655:dbl)  [unwired: 4 in]
                    n218 = call "Ackermann_Steer_Velociy_Cal.vi"("속도(mps)"=w664, "조향각(Deg)"=w663, "윤거W(m)"=w665, "축거L(m)"=w666) -> ("속도_RL(mps)"=w659:dbl, "속도_RR(mps)"=w660:dbl, "속도_FL(mps)"=w661:dbl, "속도_FR(mps)"=w662:dbl)  [unwired: 4 in]
                  }
                  frame True {
                    w667 = 0.0 ("y")
                  }
                }
                n219 = expression code="9.09*x+1600"(w644) -> (w654:dbl)
                n220 = expression code="9.09*x+1640"(w643) -> (w653:dbl)
                n221 = expression code="-8.18*x+1600"(w642) -> (w652:dbl)
                n222 = expression code="-8.18*x+1450"(w641) -> (w651:dbl)
              }
              frame 1 {
                # "-8.63*x+1590"
                # "Ackerman\nSteering 수식"
                # "-22~22deg 기준 \n각 서보 출력값의 직선방정식"
                # "전/후륜 제어"
                n223 = Equal To 0?(x=w671) -> (x = 0?=w672:bool)
                n224 = case shown="거짓" w672 {
                  tunnel: w681 -> [w697 w699]
                  tunnel: w671 -> [w696 _]
                  tunnel: [w692 w699] -> w677
                  tunnel: [w694 w699] -> w680
                  tunnel: [w693 w699] -> w678
                  tunnel: [w695 w699] -> w679
                  tunnel: [w690 w698] -> w676
                  tunnel: [w691 w698] -> w675
                  tunnel: [w688 w698] -> w674
                  tunnel: [w689 w698] -> w673
                  tunnel: w670 -> [w687 _]
                  tunnel: w669 -> [w686 _]
                  frame False {
                    n225 = call "4WIS_Steer_Angle_Cal.vi"("축거L(m)"=w687, "윤거W(m)"=w686, "조향각(deg)"=w696) -> ("FR_조향각(deg)"=w691:dbl, "FL_조향각(deg)"=w690:dbl, "RR_조향각(deg)"=w689:dbl, "RL_조향각(deg)"=w688:dbl)  [unwired: 4 in]
                    n226 = call "4WIS_Steer_Velociy_Cal.vi"("속도(mps)"=w697, "조향각(Deg)"=w696, "윤거W(m)"=w686, "축거L(m)"=w687) -> ("속도_RL(mps)"=w692:dbl, "속도_RR(mps)"=w693:dbl, "속도_FL(mps)"=w694:dbl, "속도_FR(mps)"=w695:dbl)  [unwired: 4 in]
                  }
                  frame True {
                    w698 = 0.0
                  }
                }
                n227 = expression code="9.09*x+1600"(w676) -> (w685:dbl)
                n228 = expression code="9.09*x+1640"(w675) -> (w684:dbl)
                n229 = expression code="-8.18*x+1600"(w674) -> (w683:dbl)
                n230 = expression code="-8.18*x+1450"(w673) -> (w682:dbl)
              }
              frame 2 {
                # "39.5deg"
                # "Pivot"
                n231 = Negate(x=w701) -> (-x=w702:dbl)
                n232 = Negate(x=w701) -> (-x=w700:dbl)
              }
            }
            n233 = To Word Integer(number=w599) -> (16bit integer=w603:i16)
            n234 = To Word Integer(number=w597) -> (16bit integer=w594:i16)
            n235 = To Word Integer(number=w596) -> (16bit integer=w593:i16)
            n236 = To Word Integer(number=w595) -> (16bit integer=w592:i16)
            n237 = To Word Integer(number=w591) -> (16bit integer=w587:i16)
            n238 = To Word Integer(number=w590) -> (16bit integer=w586:i16)
            n239 = To Word Integer(number=w589) -> (16bit integer=w585:i16)
            n240 = To Word Integer(number=w588) -> (16bit integer=w584:i16)
          }
          frame True {
            # "FL_M\nFR_M\nRR_M\nRL_M"
            # "FL_S\nFR_S\nRL_S\nRR_S"
            # "Auto"
            n241 = Build Array(w731, w730) -> (w729:bool[])
            n242 = Boolean Array To Number(Boolean array=w729) -> (number=w728:u32)
            n243 = case shown="1" w728 {
              tunnel: w727 -> [_ w749 _ _]
              tunnel: w726 -> [_ w748 _ _]
              tunnel: w721 -> [_ w747 _ _]
              tunnel: [1600.0 w746 1600.0 1600.0] -> w713
              tunnel: [1640.0 w745 1640.0 1640.0] -> w712
              tunnel: [1600.0 w744 1600.0 1600.0] -> w711
              tunnel: [1450.0 w743 1450.0 1450.0] -> w710
              tunnel: [w736 w742 w839 w840] -> w709
              tunnel: [w736 w741 w839 w840] -> w716
              tunnel: [w736 w740 w839 w840] -> w715
              tunnel: [w736 w739 w839 w840] -> w714
              tunnel: w707 -> [_ w738 _ _]
              tunnel: w708 -> [_ w737 _ _]
              frame 0, Default {
                w736 = 0.0
                # "H_M : Auto Fail"
              }
              frame 1 {
                # "H_A : Normal"
                n244 = case shown="1" w747 {
                  tunnel: w749 -> [w770 w807 w825]
                  tunnel: w748 -> [w764 w801 _]
                  tunnel: [w768 w805 1940.0] -> w746
                  tunnel: [w767 w804 1320.0] -> w745
                  tunnel: [w766 w803 1300.0] -> w744
                  tunnel: [w765 w802 1950.0] -> w743
                  tunnel: [w755 w790 w828] -> w742
                  tunnel: [w754 w794 w830] -> w741
                  tunnel: [w753 w795 w829] -> w740
                  tunnel: [w752 w791 w828] -> w739
                  tunnel: w738 -> [w751 w788 _]
                  tunnel: w737 -> [w750 w787 _]
                  frame 0, Default {
                    # "0:전륜 조향모드"
                    n245 = To Double Precision Float(number=w764) -> (double precision float=w761:dbl)
                    n246 = In Range and Coerce(upper limit=i16 48, x=w770, lower limit=i16 -49) -> (coerced(x)=w769:i16)  [unwired: 1 out]
                    n247 = To Double Precision Float(number=w769) -> (double precision float=w763:dbl)
                    n248 = Equal?(x=w761, y=0.0) -> (x = y?=w760:bool)
                    n249 = case shown="참" w760 {
                      tunnel: w761 -> [w783 _]
                      tunnel: [w780 w786] -> w754
                      tunnel: [w779 w786] -> w755
                      tunnel: [w778 w786] -> w753
                      tunnel: [w777 w786] -> w752
                      tunnel: [w775 w785] -> w759
                      tunnel: [w776 w785] -> w758
                      tunnel: [w773 w785] -> w757
                      tunnel: [w774 w785] -> w756
                      tunnel: w763 -> [w784 w786]
                      tunnel: w751 -> [w782 _]
                      tunnel: w750 -> [w781 _]
                      frame False {
                        n250 = call "Ackermann_Steer_Angle_Cal.vi"("축거L(m)"=w782, "윤거W(m)"=w781, "조향각(deg)"=w783) -> ("FR_조향각(deg)"=w776:dbl, "FL_조향각(deg)"=w775:dbl, "RR_조향각(deg)"=w774:dbl, "RL_조향각(deg)"=w773:dbl)  [unwired: 4 in]
                        n251 = call "Ackermann_Steer_Velociy_Cal.vi"("속도(mps)"=w784, "조향각(Deg)"=w783, "윤거W(m)"=w781, "축거L(m)"=w782) -> ("속도_RL(mps)"=w777:dbl, "속도_RR(mps)"=w778:dbl, "속도_FL(mps)"=w779:dbl, "속도_FR(mps)"=w780:dbl)  [unwired: 4 in]
                      }
                      frame True {
                        w785 = 0.0 ("y")
                      }
                    }
                    n252 = expression code="9.09*x+1600"(w759) -> (w768:dbl)
                    n253 = expression code="9.09*x+1640"(w758) -> (w767:dbl)
                    n254 = expression code="-8.18*x+1600"(w757) -> (w766:dbl)
                    n255 = expression code="-8.18*x+1450"(w756) -> (w765:dbl)
                  }
                  frame 1 {
                    # "1:전/후륜 조향모드"
                    n256 = To Double Precision Float(number=w801) -> (double precision float=w798:dbl)
                    n257 = Equal?(x=w798, y=0.0) -> (x = y?=w799:bool)
                    n258 = In Range and Coerce(upper limit=i16 48, x=w807, lower limit=i16 -49) -> (coerced(x)=w806:i16)  [unwired: 1 out]
                    n259 = To Double Precision Float(number=w806) -> (double precision float=w797:dbl)
                    n260 = case shown="거짓" w799 {
                      tunnel: w797 -> [w821 w823]
                      tunnel: w798 -> [w820 _]
                      tunnel: [w814 w823] -> w791
                      tunnel: [w817 w823] -> w790
                      tunnel: [w815 w823] -> w795
                      tunnel: [w816 w823] -> w794
                      tunnel: [w812 w822] -> w792
                      tunnel: [w813 w822] -> w789
                      tunnel: [w810 w822] -> w793
                      tunnel: [w811 w822] -> w796
                      tunnel: w788 -> [w819 _]
                      tunnel: w787 -> [w818 _]
                      frame False {
                        n261 = call "4WIS_Steer_Velociy_Cal.vi"("속도(mps)"=w821, "조향각(Deg)"=w820, "윤거W(m)"=w818, "축거L(m)"=w819) -> ("속도_RL(mps)"=w814:dbl, "속도_RR(mps)"=w815:dbl, "속도_FL(mps)"=w817:dbl, "속도_FR(mps)"=w816:dbl)  [unwired: 4 in]
                        n262 = call "4WIS_Steer_Angle_Cal.vi"("축거L(m)"=w819, "윤거W(m)"=w818, "조향각(deg)"=w820) -> ("FR_조향각(deg)"=w813:dbl, "FL_조향각(deg)"=w812:dbl, "RR_조향각(deg)"=w811:dbl, "RL_조향각(deg)"=w810:dbl)  [unwired: 4 in]
                      }
                      frame True {
                        w822 = 0.0
                      }
                    }
                    n263 = expression code="9.09*x+1600"(w792) -> (w805:dbl)
                    n264 = expression code="9.09*x+1640"(w789) -> (w804:dbl)
                    n265 = expression code="-8.18*x+1600"(w793) -> (w803:dbl)
                    n266 = expression code="-8.18*x+1450"(w796) -> (w802:dbl)
                  }
                  frame 2 {
                    # "CCW"
                    # "2: Pivot"
                    n267 = In Range and Coerce(upper limit=i16 20, x=w825, lower limit=i16 -21) -> (coerced(x)=w824:i16)  [unwired: 1 out]
                    n268 = To Double Precision Float(number=w824) -> (double precision float=w828:dbl)
                    n269 = Negate(x=w828) -> (-x=w830:dbl)
                    n270 = Negate(x=w828) -> (-x=w829:dbl)
                  }
                }
              }
              frame 2 {
                w839 = 0.0
              }
              frame 3 {
                w840 = 0.0
              }
            }
            n271 = To Word Integer(number=w709) -> (16bit integer=w720:i16)
            n272 = To Word Integer(number=w716) -> (16bit integer=w719:i16)
            n273 = To Word Integer(number=w715) -> (16bit integer=w718:i16)
            n274 = To Word Integer(number=w714) -> (16bit integer=w717:i16)
            n275 = To Word Integer(number=w713) -> (16bit integer=w725:i16)
            n276 = To Word Integer(number=w712) -> (16bit integer=w724:i16)
            n277 = To Word Integer(number=w711) -> (16bit integer=w723:i16)
            n278 = To Word Integer(number=w710) -> (16bit integer=w722:i16)
          }
        }
      }
      frame True {
        w856 = i16 0
        # "E-Stop"
        n279 = To Word Integer(number=1600.0) -> (16bit integer=w855:i16)
        n280 = To Word Integer(number=1620.0) -> (16bit integer=w854:i16)
        n281 = To Word Integer(number=1620.0) -> (16bit integer=w853:i16)
        n282 = To Word Integer(number=1590.0) -> (16bit integer=w852:i16)
      }
    }
    "FL_Steer_Feed" <- w475
    "FR_Steer_Feed" <- w474
    "RL_Steer_Feed" <- w473
    "RR_Steer_Feed" <- w472
    n283 = In Range and Coerce(upper limit=i16 48, x=w471, lower limit=i16 -49) -> (coerced(x)=→"FL_RPM":i16)  [unwired: 1 out]
    n284 = In Range and Coerce(upper limit=i16 48, x=w470, lower limit=i16 -49) -> (coerced(x)=→"FR_RPM":i16)  [unwired: 1 out]
    n285 = In Range and Coerce(upper limit=i16 48, x=w469, lower limit=i16 -49) -> (coerced(x)=→"RR_RPM":i16)  [unwired: 1 out]
    n286 = In Range and Coerce(upper limit=i16 48, x=w468, lower limit=i16 -49) -> (coerced(x)=→"RL_RPM":i16)  [unwired: 1 out]
    n287 = In Range and Coerce(upper limit=i16 1950, x=w475, lower limit=i16 1350) -> (coerced(x)=w523:i16)  [unwired: 1 out]
    n288 = In Range and Coerce(upper limit=i16 1850, x=w474, lower limit=i16 1300) -> (coerced(x)=w516:i16)  [unwired: 1 out]
    n289 = In Range and Coerce(upper limit=i16 1850, x=w473, lower limit=i16 1300) -> (coerced(x)=w515:i16)  [unwired: 1 out]
    n290 = In Range and Coerce(upper limit=i16 1950, x=w472, lower limit=i16 1200) -> (coerced(x)=w514:i16)  [unwired: 1 out]
    n291 = xnode "읽기/쓰기 컨트롤"("FPGA VI 참조 입력"=w533, "에러 입력"=w532, "FL_Steer"=w523, "FR_Steer"=w516, "RL_Steer"=w515, "RR_Steer"=w514) -> ("FPGA VI 참조 출력"=w538:refnum<k20>, "에러 출력"=w537:errorcluster)
    n292 = local read "정지"() -> (w536:bool)
    n293 = local read "K_ZERO_CMD"() -> (w499:T1)
  }
  n294 = while {
    tunnel: w22 -> [w869]
    tunnel: w23 -> [w870]
    shift-right: [w864] -> _
    shift-left: w24 -> [w862]
    shift-right: [w863] -> _
    shift-left: FALSE -> [w861]
    tunnel: [w859] -> w26
    tunnel: [w858] -> w27
    shift-right: [w857] -> _
    shift-left: w20 -> [w867]
    stop <- w860 stop-if-true
    # "UDP Receive Loop"
    n295 = Wait Until Next ms Multiple(millisecond multiple=u32 50 ("milliseconds to wait")) -> ()  [unwired: 1 out]
    n296 = UDP Read(connection ID=w869, timeout ms (25000)=100, 8:w870) -> (data out=w865:string, error out=w866:errorcluster, 3:w868:refnum<k16>)  [unwired: 1 in, 2 out]
    n297 = case shown="에러 없음" w866 {
      selector: w866 -> [w875 w881]
      tunnel: w868 -> [w874 w882]
      tunnel: w867 -> [w878 w880]
      tunnel: w865 -> [w879 _]
      tunnel: [w877 w885] -> w864
      tunnel: [w876 w883] -> w863
      tunnel: w862 -> [_ w885]
      tunnel: w861 -> [_ w884]
      tunnel: [w874 w882] -> w859
      tunnel: [w875 w881] -> w858
      tunnel: [w873 w880] -> w857
      frame No Error {
        n298 = Type Cast(type=w878, x=w879) -> (*(type *) &x=w873:T1)
        n299 = local read "Re_M/A"() -> (w876:bool)
        n300 = Tick Count (ms)() -> (millisecond timer value=w877:u32)
      }
      frame Error {
        n301 = Tick Count (ms)() -> (millisecond timer value=w886:u32)
        n302 = Subtract(x=w886, y=w885) -> (x-y=w887:u32)
        n303 = Greater?(x=w887, y=u32 1500) -> (0:w889:bool)
        n304 = Select(t=FALSE, s=w889, f=w884) -> (s? t:f=w883:bool)
      }
    }
    "K_ZERO_CMD" <- w857
    n305 = local read "정지"() -> (w860:bool)
  }
  n306 = UDP Close(connection ID=w26, 8:w27) -> (error out=w11:errorcluster)  [unwired: 1 out]
  n307 = UDP Close(connection ID=w18, 8:w19) -> (error out=w10:errorcluster)  [unwired: 1 out]
  n308 = VISA Flush I/O Buffer(VISA resource name=w38, error in (no error)=w39) -> (VISA resource name out=w40:refnum<visa-resource-name>, error out=w41:errorcluster)  [unwired: 1 in]
  n309 = VISA Flush I/O Buffer(VISA resource name=w49, error in (no error)=w48) -> (VISA resource name out=w47:refnum<visa-resource-name>, error out=w46:errorcluster)  [unwired: 1 in]
  n310 = VISA Close(VISA resource name=w40, error in (no error)=w41) -> (error out=w9:errorcluster)
  n311 = VISA Close(VISA resource name=w47, error in (no error)=w46) -> (error out=w8:errorcluster)
  n312 = Merge Errors(w11, w10, w7, w9, w8) -> (w5:errorcluster)
  n313 = xnode "Close FPGA VI Reference"("FPGA VI 참조 입력"=w6, "에러 입력"=w5) -> ()  [unwired: 1 out]
